vi "DataLogging.vi"(4 "Tab?":bool, 6 "New Line?":bool, 7 "Name":string, 8 "error in (no error)":errorcluster, 10 "WriteToFile?":bool, 11 "Variant In":variant) -> (0 "error out":errorcluster, 3 "FinalText":string)   [LabVIEW 2017]
uses:
  <vilib>/Utility/Data Type/Type Definitions/Data Type.ctl
  <vilib>/Utility/Data Type/NI_Data Type.lvlib
panel:
  out "Type":T1
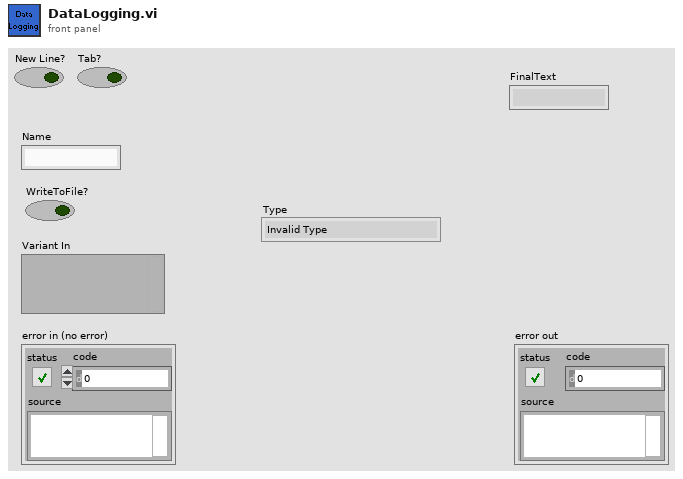
[diagram p1: front panel]
types:
  T1 = typedef "NI_Data Type.lvlib/Data Type.ctl" = enum8{"Invalid Type", "Void", "I8", "I16", "I32", "I64", "U8", "U16", "U32", "U64", "Single Float", "Double Float", "Extended Float", "Single Complex", "Double Complex", "Extended Complex", "Enum U8", "Enum U16", "Enum U32", "Enum U64", "Single Float With Unit", "Double Float With Unit", "Extended Float With Unit", "Single Complex with Unit", "Double Complex with Unit", "Extended Complex with Unit", "Boolean", "String", "Path", "Picture", "Tag", "Array", "Cluster", "Variant", "LV Variant", "Waveform", "Timestamp", "Digital Waveform", "Digital Data", "ExpressData", "Refnum", "External Data", "VI", "Poly VI", "LabVIEW Class Instance", "Fixed Point"}
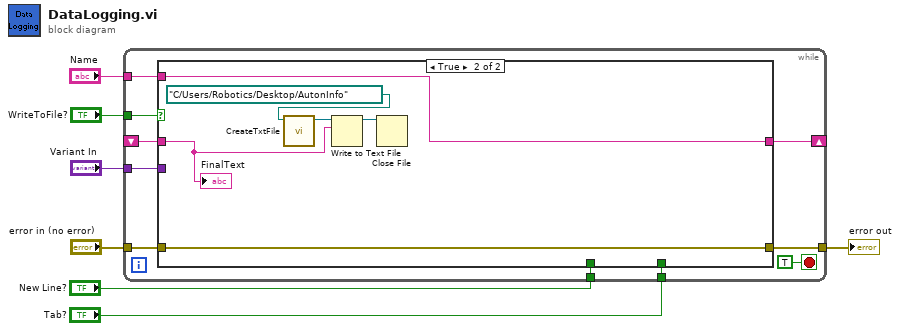
[diagram p0: block diagram]
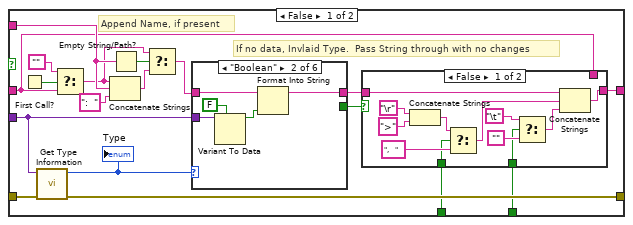
[diagram p2: hidden frame]
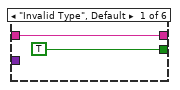
[diagram p4: hidden frame]
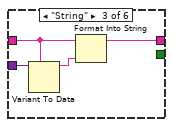
[diagram p5: hidden frame]
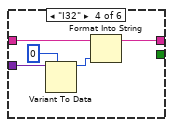
[diagram p6: hidden frame]
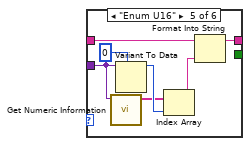
[diagram p7: hidden frame]
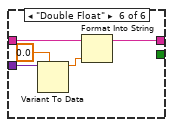
[diagram p8: hidden frame]
diagram:
  n1 = while {
    tunnel: "Variant In" -> [w17]
    shift-right: [w10] -> _
    shift-left: _ -> [w13]
    tunnel: "WriteToFile?" -> [w8]
    tunnel: "error in (no error)" -> [w15]
    tunnel: [w14] -> w4
    tunnel: "Name" -> [w12]
    tunnel: "New Line?" -> [w11]
    tunnel: "Tab?" -> [w9]
    stop <- TRUE stop-if-true
    n2 = case shown="True" w8 {
      tunnel: w17 -> [w35 _]
      tunnel: w15 -> [w34 w82]
      tunnel: [w33 w82] -> w14
      tunnel: w13 -> [w18 w78]
      tunnel: w12 -> [w29 w81]
      tunnel: w11 -> [w24 _]
      tunnel: [w19 w81] -> w10
      tunnel: w9 -> [w22 _]
      frame False {
        # "If no data, Invlaid Type.  Pass String through with no changes"
        # "Append Name, if present"
        n3 = First Call?() -> (First Call?: T/F=w31:bool)
        n4 = call <vilib>:"Get Type Information.vi"("error in (no error)"=w34, "Variant"=w35) -> ("error out"=w33:errorcluster, "Type"=w21:T1)  [unwired: 5 in, 3 out]
        "Type" <- w21
        n5 = Select(t="", s=w31, f=w18) -> (s? t:f=w26:string)
        n6 = Concatenate Strings(w26, w29, ":  " ("string")) -> (w27:string)
        n7 = Empty String/Path?(string/path=w29) -> (empty?=w30:bool)
        n8 = Select(t=w26, s=w30, f=w27) -> (s? t:f=w28:string)
        n9 = case shown="\"Boolean\"" w21 {
          tunnel: w35 -> [_ w55 w59 w64 w67 w74]
          tunnel: [w50 w52 w57 w62 w71 w76] -> w23
          tunnel: w28 -> [w50 w51 w56 w61 w70 w75]
          tunnel: [TRUE _ _ _ _ _] -> w20
          frame "Invalid Type", Default {
          }
          frame "Boolean" {
            n10 = Variant To Data(type=FALSE, Variant=w55) -> (data=w53:bool)  [unwired: 1 in, 1 out]
            n11 = Format Into String(initial string=w51, w53) -> (resulting string=w52:string)  [unwired: 2 in, 1 out]
          }
          frame "String" {
            n12 = Variant To Data(type=w56, Variant=w59) -> (data=w58:string)  [unwired: 1 in, 1 out]
            n13 = Format Into String(initial string=w56, w58) -> (resulting string=w57:string)  [unwired: 2 in, 1 out]
          }
          frame "I32" {
            n14 = Variant To Data(type=0, Variant=w64) -> (data=w63:i32)  [unwired: 1 in, 1 out]
            n15 = Format Into String(initial string=w61, w63) -> (resulting string=w62:string)  [unwired: 2 in, 1 out]
          }
          frame "Enum U16" {
            n16 = call <vilib>:"Get Numeric Information.vi"("Variant"=w67) -> ("Enum Names"=w68:string[])  [unwired: 7 in, 3 out]
            n17 = Variant To Data(type=0, Variant=w67) -> (data=w69:i32)  [unwired: 1 in, 1 out]
            n18 = Index Array(array=w68, index=w69) -> (element=w66:string)
            n19 = Format Into String(initial string=w70, w66) -> (resulting string=w71:string)  [unwired: 2 in, 1 out]
          }
          frame "Double Float" {
            n20 = Variant To Data(type=0.0, Variant=w74) -> (data=w72:dbl)  [unwired: 1 in, 1 out]
            n21 = Format Into String(initial string=w75, w72) -> (resulting string=w76:string)  [unwired: 2 in, 1 out]
          }
        }
        n22 = case shown="False" w20 {
          tunnel: w24 -> [w44 _]
          tunnel: w23 -> [w43 _]
          tunnel: w22 -> [w37 _]
          tunnel: [w36 w48] -> w19
          tunnel: w18 -> [_ w48]
          frame False {
            n23 = Concatenate Strings("\r", ">") -> (w45:string)
            n24 = Select(t=w45, s=w44, f=",   ") -> (s? t:f=w42:string)
            n25 = Select(t="\t", s=w37, f="") -> (s? t:f=w40:string)
            n26 = Concatenate Strings(w43, w42, w40) -> (w36:string)
          }
          frame True {
          }
        }
      }
      frame True {
        n27 = call "CreateTxtFile.vi"("pathIn"=path "C:/Users/Robotics/Desktop/AutonInfo") -> ("refnumOut"=w79:refnum<file>)  [unwired: 10 in]
        n28 = Write to Text File(file (use dialog)=w79, text=w78) -> (refnum out=w80:refnum<file>)  [unwired: 2 in, 2 out]
        n29 = Close File(refnum=w80) -> ()  [unwired: 1 in, 2 out]
        "FinalText" <- w78
      }
    }
  }
  "error out" <- w4
